vi "Compile Channel Groups.vi"(8 "error in":errorcluster, 11 "Settings(JSON)":string) -> (0 "error out":errorcluster, 3 "ChannelGroups":T1)   [LabVIEW 2026, in "Template Deployment Hooks.lvlib"]
uses:
  Template Deployment Hooks.lvlib
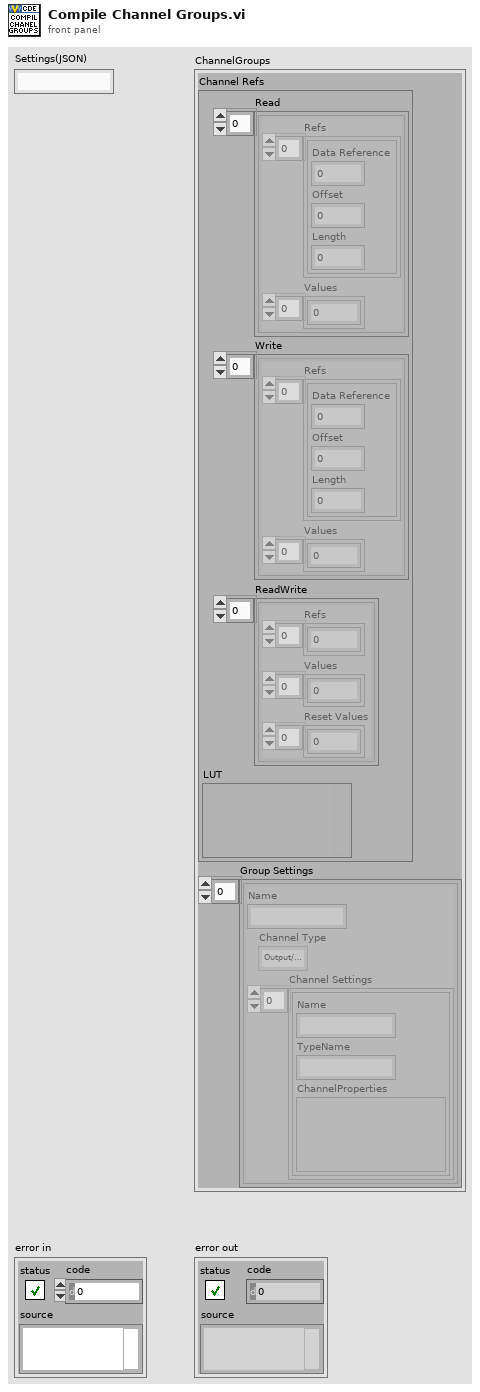
[diagram p1: front panel]
types:
  T1 = cluster{"Channel Refs":cluster{"Read":cluster{"Refs":cluster{"Data Reference":i32, "Offset":u64, "Length":u64}[], "Values":dbl[]}[], "Write":cluster{"Refs":cluster{"Data Reference":i32, "Offset":u64, "Length":u64}[], "Values":dbl[]}[], "ReadWrite":cluster{"Refs":i32[], "Values":dbl[], "Reset Values":dbl[]}[], "LUT":variant}, "Group Settings":cluster{"Name":string, "Channel Type":enum16{"Output/Write", "Input/Read", "Input/ReadWrite"}, "Channel Settings":cluster{"Name":string, "TypeName":string, "ChannelProperties":variant}[]}[]}
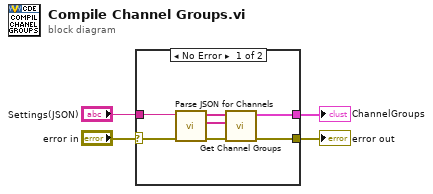
[diagram p0: block diagram]
diagram:
  n1 = case shown="No Error" "error in" {
    selector: "error in" -> [w11 w12]
    tunnel: [w10 w12] -> w4
    tunnel: "Settings(JSON)" -> [w9 _]
    tunnel: [w8 _] -> w1
    frame No Error {
      n2 = call "Parse JSON for Channels.vi"("error in"=w11, "JSON"=w9) -> ("error out"=w7:errorcluster, "Channel JSON List"=w5:string[], "Channel Type List"=w6:string[])  [unwired: 7 in]
      n3 = call "Get Channel Groups.vi"("error in"=w7, "Channel JSON List"=w5, "Channel Type List"=w6) -> ("error out"=w10:errorcluster, "ChannelGroups"=w8:T1)  [unwired: 7 in]
    }
    frame Error {
    }
  }
  "error out" <- w4
  "ChannelGroups" <- w1
